vi "Ramp Drive Speed.vi"(10 "Ramp Value":dbl, 11 "New":dbl) -> (3 "Output":dbl)   [LabVIEW 2012]
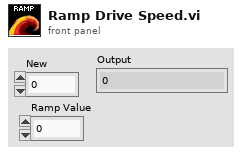
[diagram p1: front panel]
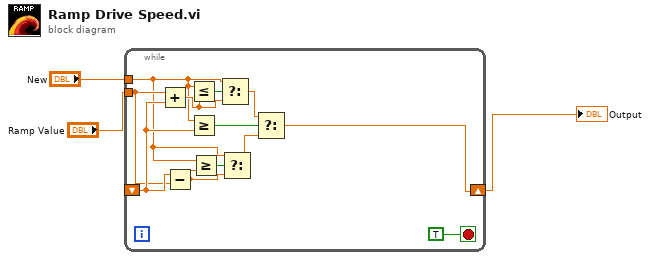
[diagram p0: block diagram]
diagram:
  n1 = while {
    tunnel: "New" -> [w7]
    shift-right: [w5] -> w2
    shift-left: _ -> [w9]
    tunnel: "Ramp Value" -> [w8]
    stop <- TRUE stop-if-true
    n2 = Add(x=w8, y=w9) -> (x+y=w12:dbl)
    n3 = Subtract(x=w9, y=w8) -> (x-y=w6:dbl)
    n4 = Less Or Equal?(x=w7, y=w12) -> (x <= y?=w13:bool)
    n5 = Greater Or Equal?(x=w7, y=w9) -> (x >= y?=w15:bool)
    n6 = Greater Or Equal?(x=w7, y=w6) -> (x >= y?=w10:bool)
    n7 = Select(t=w7, s=w13, f=w12) -> (s? t:f=w14:dbl)
    n8 = Select(t=w7, s=w10, f=w6) -> (s? t:f=w11:dbl)
    n9 = Select(t=w14, s=w15, f=w11) -> (s? t:f=w5:dbl)
  }
  "Output" <- w2
